vi "Pane Resize.vi"(8 "error in (no error)":errorcluster, 10 "NewBnds":T1, 11 "Terminal in":refnum<class "Terminal.lvclass">) -> (0 "error out":errorcluster, 3 "Terminal out":refnum<class "Terminal.lvclass">)   [LabVIEW 2020, in "Terminal.lvlib" / "Terminal.lvclass"]
uses:
  Terminal.lvclass
  <vilib>/Utility/miscctls.llb/LVRectTypeDef.ctl
  <vilib>/Utility/miscctls.llb/LVBoundsTypeDef.ctl
  Terminal.lvclass/Terminal.ctl
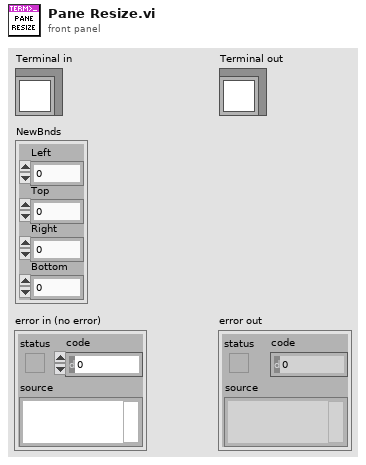
[diagram p1: front panel]
types:
  T1 = typedef "LVRectTypeDef.ctl" = cluster{"Left":i16, "Top":i16, "Right":i16, "Bottom":i16}
  T2 = typedef "LVBoundsTypeDef.ctl" = cluster{"Width":u32, "Height":u32}
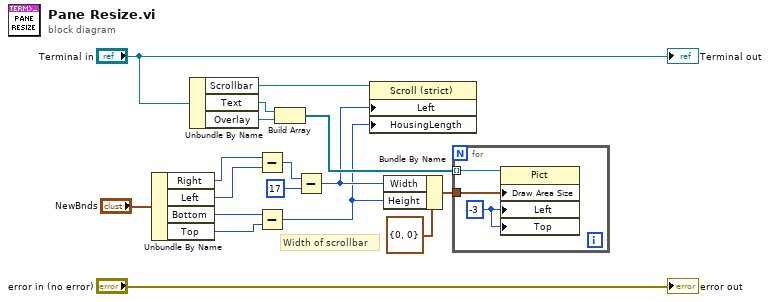
[diagram p0: block diagram]
diagram:
  # "Width of scrollbar"
  n1 = Unbundle By Name("NewBnds") -> ("Right"=w15:i16, "Left"=w14:i16, "Bottom"=w13:i16, "Top"=w12:i16)
  n2 = Unbundle By Name("Terminal in") -> ("Scrollbar"=w9:refnum<vi>, "Text"=w8:refnum<vi>, "Overlay"=w7:refnum<vi>)
  n3 = Subtract(x=w15, y=w14) -> (x-y=w11:i16)
  n4 = Subtract(x=w13, y=w12) -> (x-y=w3:i16)
  n5 = Build Array(w8, w7) -> (w6:refnum<vi>[])
  n6 = Subtract(x=w11, y=i16 17) -> (x-y=w4:i16)
  n7 = property class="Scroll (strict)"(reference=w9, "Left"=w4, "HousingLength"=w3) -> ()  [unwired: 1 in, 2 out]
  n8 = Bundle By Name(cluster=T2 {"Width"=0, "Height"=0} ("Draw Area Size"), "Width"=w4, "Height"=w3) -> (w2:T2)
  n9 = for {
    tunnel: w6 -> [w20] mode=indexing
    tunnel: w2 -> [w19]
    w18 = -3 ("Position:Left")
    n10 = property class="Pict"(reference=w20, "Draw Area Size"=w19, "Left"=w18, "Top"=w18) -> ()  [unwired: 1 in, 2 out]
  }
  "error out" <- "error in (no error)"
  "Terminal out" <- "Terminal in"
